vi "Telnet Write Filter.vi"(1 "Data":string) -> (0 "Data out":string)   [LabVIEW 2014]
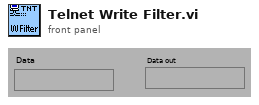
[diagram p1: front panel]
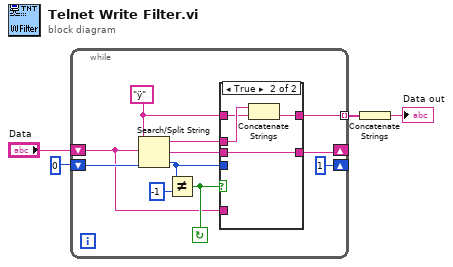
[diagram p0: block diagram]
diagram:
  n1 = while {
    tunnel: [w6] -> w2 mode=indexing
    shift-left: "Data" -> [w9]
    shift-right: [w10] -> _
    shift-left: 0 -> [w15]
    shift-right: [1] -> _
    stop <- w12 continue-if-true
    w7 = "ÿ" ("regular expression")
    n2 = Search/Split String(string=w9, search string/char (-)=w7, offset (0)=w15) -> (substring before match=w8:string, match + rest of string=w14:string, offset of match=w11:i32)
    n3 = Not Equal?(x=w11, y=-1) -> (x != y?=w12:bool)
    n4 = case shown="True" w12 {
      tunnel: w14 -> [_ w18]
      tunnel: w8 -> [w16 w21]
      tunnel: [w17 w18] -> w10
      tunnel: w9 -> [w17 _]
      tunnel: w11 -> [_ _]
      tunnel: w7 -> [_ w20]
      tunnel: [w16 w19] -> w6
      frame False {
      }
      frame True {
        n5 = Concatenate Strings(w21, w20) -> (w19:string)
      }
    }
  }
  n6 = Concatenate Strings(w2) -> (→"Data out":string)
